vi "Host-Version-Top-Level.vi"() -> ()   [LabVIEW 2015]
uses:
  SETI_LV/SETI_LV.lvlib
panel:
  out "Errors":cluster{"lower limit":sgl, "Index":i32}[](array[cluster])
  out "ChirpedData (out)":csg[](array[numeric])
  out "Fft Results (out)":csg[](array[numeric])
  out "Expected\nPower Spectrum":sgl[](array[numeric])
  out "Calculated\nPower Spectrum":sgl[](array[numeric])
  in  "Max Error":sgl=0.0001
  out "Results\nMatch?":bool
  in  "Run #\nto Load":i32=1
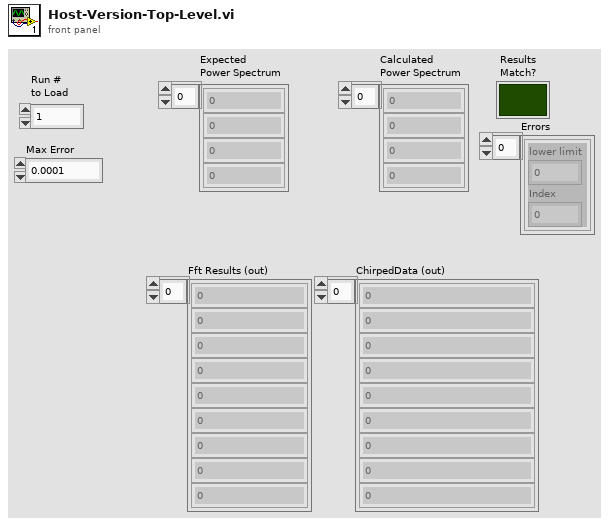
[diagram p1: front panel]
types:
  T1 = typedef "SETI_LV.lvlib/ChirpFFT Pairs.ctl" = cluster{"Chirp/Fft Pair 1 - Chirp Rate":dbl, "Chirp/Fft Pair 1 - Chirp Rate Ind":i32, "Chirp/Fft Pair 1 - Fft Length":i32, "Chirp/Fft Pair 1 - Pulse Find":i32, "Chirp/Fft Pair 1 - Gauss Fit":i32}
  T2 = typedef "SETI_LV.lvlib/Power Spectrum Data.ctl" = cluster{"icfft":i32, "NumDataPoints":i32, "Power Spectrum":sgl[]}
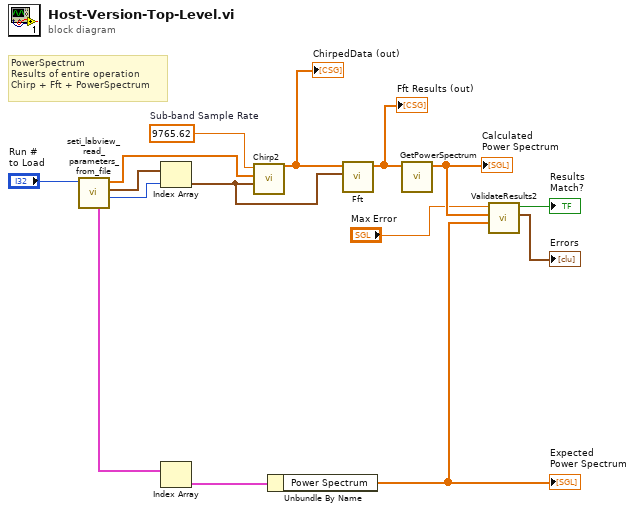
[diagram p0: block diagram]
diagram:
  w12 = 9765.62  # Sub-band Sample Rate
  # "PowerSpectrum\nResults of entire operation\nChirp + Fft + PowerSpectrum"
  n1 = call "seti_labview_read_parameters_from_file.vi"("Run Number\nto Load"="Run #\nto Load") -> ("start_icfft"=w6:i32, "Chirp FFT Pairs"=w13:T1[], "Data Points (Source)"=w11:csg[], "Array of Power Spectrum Data\n(Expected Results)"=w14:T2[])  [unwired: 4 in, 3 out]
  n2 = Index Array(array=w13, index=w6) -> (element=w9:T1)
  n3 = Index Array(array=w14) -> (element=w7:T2)  [unwired: 1 in]
  n4 = call "Chirp2.vi"("Chirp Parameters (in)"=w9, "DataPoints (in)"=w11, "Sub-band Sample Rate (in)"=w12) -> ("ChirpedData (out)"=w10:csg[])  [unwired: 8 in]
  "ChirpedData (out)" <- w10
  n5 = Unbundle By Name(w7) -> ("Power Spectrum"=w4:sgl[])
  "Expected\nPower Spectrum" <- w4
  n6 = call "Fft.vi"("Chirp Parameters (in)"=w9, "DataPoints (in)"=w10) -> ("Fft Results (out)"=w8:csg[])  [unwired: 9 in]
  "Fft Results (out)" <- w8
  n7 = call "GetPowerSpectrum.vi"("Fft Results (in)"=w8) -> ("PowerSpectrum (out)"=w5:sgl[])  [unwired: 10 in]
  "Calculated\nPower Spectrum" <- w5
  n8 = call "ValidateResults2.vi"("PowerSpectrum2 (in)"=w4, "PowerSpectrum1 (in)"=w5, "Max Error"="Max Error") -> ("Errors"=→"Errors":cluster{"lower limit":sgl, "Index":i32}[], "Results Match?"=→"Results\nMatch?":bool)  [unwired: 7 in]
